vi "Results Status Update Process__core.vi"(8 "error in (no error)":errorcluster, 10 "TestRunner_UI_Refs":T2, 11 "TestStatusEvents":T1) -> (0 "error out":errorcluster)   [LabVIEW 2011, in "GraphicalTestRunner.lvlib"]
uses:
  GraphicalTestRunner.lvlib
  Classes/TestResult/resultStatus--enum.ctl
  Classes/TestSuite/suiteStatusChanged--Cluster.ctl
  Classes/TestSuite/suiteStatus--enum.ctl
  Classes/TestSuite/TestSuite.lvclass
  FailbarStatus--Enum.ctl
  Classes/TestResult/TestResult.lvclass
  <userlib>/_OpenG.lib/file/file.llb/Strip Path Extension - String__ogtk.vi
  Libraries/VITesterUtilities.lvlib
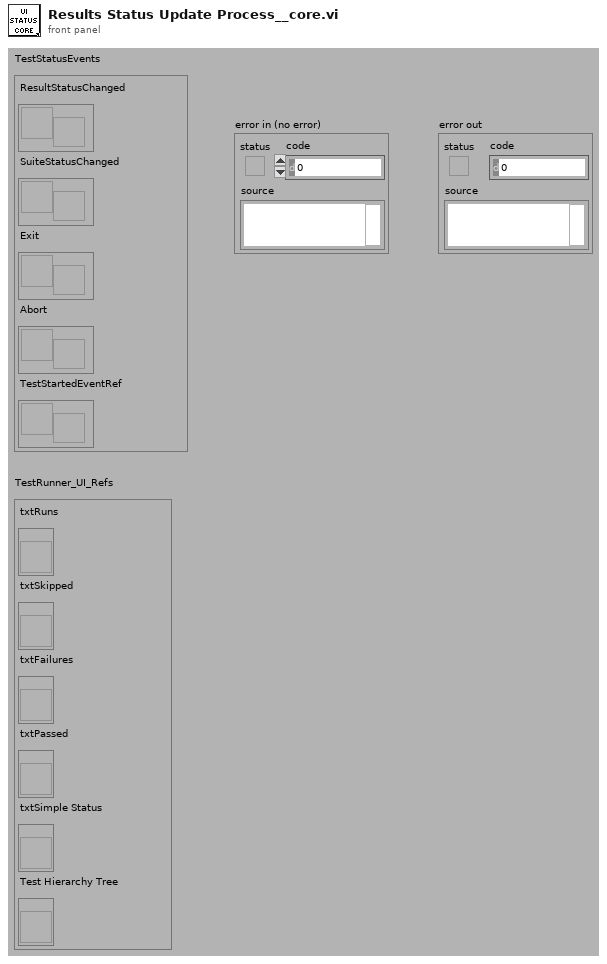
[diagram p1: front panel]
types:
  T1 = cluster{"ResultStatusChanged":refnum<user-event>, "SuiteStatusChanged":refnum<user-event>, "Exit":refnum<user-event>, "Abort":refnum<user-event>, "TestStartedEventRef":refnum<user-event>}
  T2 = cluster{"txtRuns":refnum<vi>, "txtSkipped":refnum<vi>, "txtFailures":refnum<vi>, "txtPassed":refnum<vi>, "txtSimple Status":refnum<vi>, "Test Hierarchy Tree":refnum<vi>}
  T3 = typedef "TestSuite.lvclass/suiteStatus--enum.ctl" = enum16{"suiteStart", "suiteStop", "suiteSkip"}
  T4 = typedef "GraphicalTestRunner.lvlib/FailbarStatus--Enum.ctl" = enum16{"Initialize", "Start", "Update Progress", "Fail", "Pass"}
  T5 = typedef "TestResult.lvclass/resultStatus--enum.ctl" = enum16{"testPass", "testFailure", "testError", "testSkipped"}
  T6 = typedef "TestResult.lvclass/failure.ctl" = cluster{"test":refnum<class>, "error":errorcluster}
  T7 = typedef "TestResult.lvclass/errors.ctl" = T8[]
  T8 = typedef "TestResult.lvclass/error.ctl" = cluster{"test":refnum<class>, "error":errorcluster}
  T9 = typedef "TestResult.lvclass/skipped.ctl" = T10[]
  T10 = typedef "TestResult.lvclass/skip.ctl" = cluster{"test":refnum<class>, "error":errorcluster}
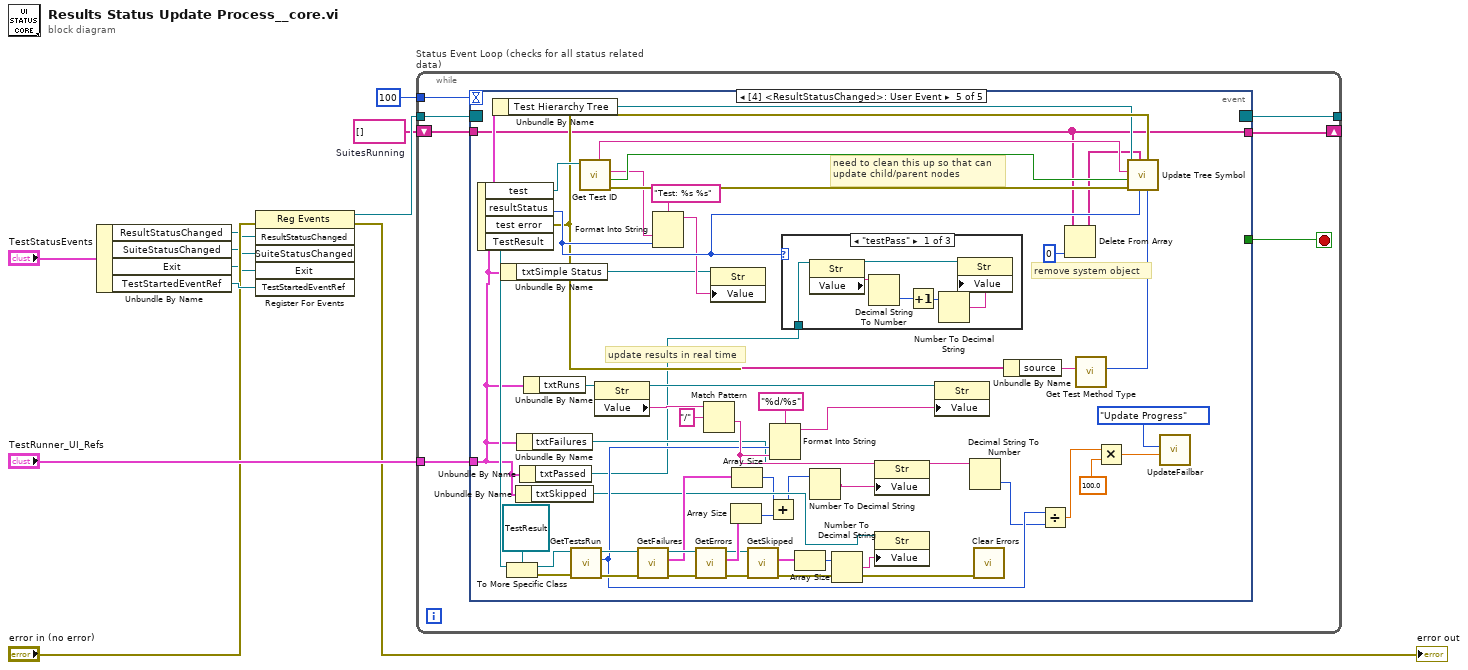
[diagram p0: block diagram]
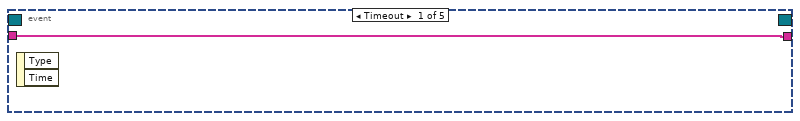
[diagram p2: hidden frame]
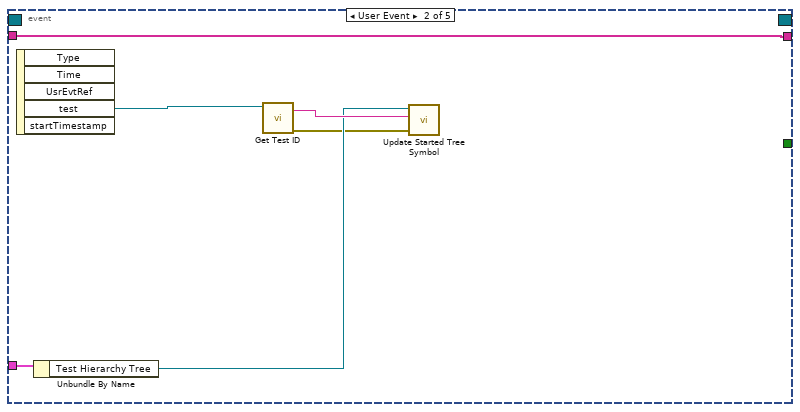
[diagram p3: hidden frame]
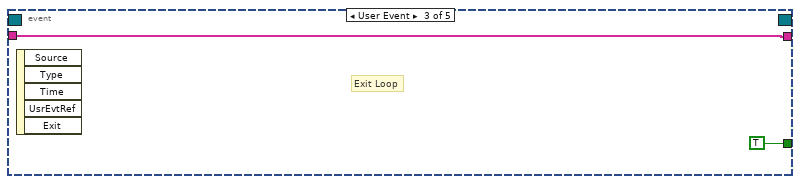
[diagram p4: hidden frame]
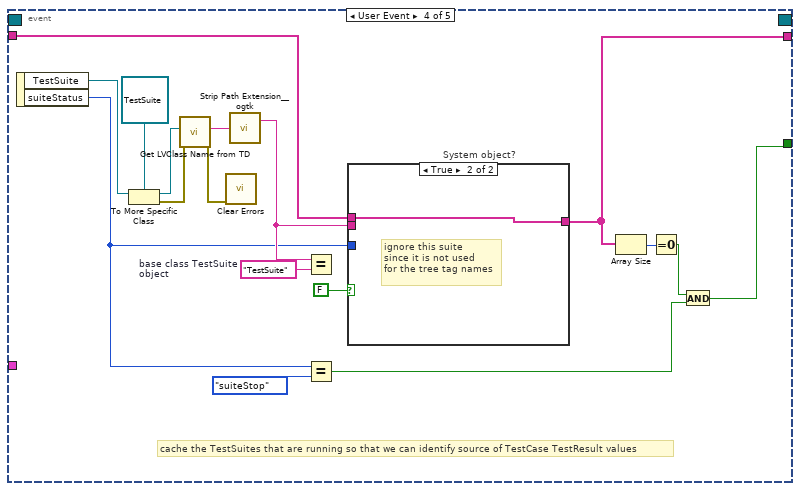
[diagram p5: hidden frame]
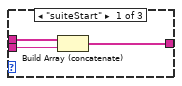
[diagram p7: hidden frame]
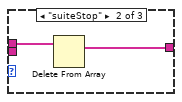
[diagram p8: hidden frame]
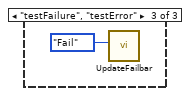
[diagram p10: hidden frame]
diagram:
  w1 = string[] []  # SuitesRunning
  n1 = Unbundle By Name("TestStatusEvents") -> ("ResultStatusChanged"=w5:refnum<user-event>, "SuiteStatusChanged"=w6:refnum<user-event>, "Exit"=w7:refnum<user-event>, "TestStartedEventRef"=w11:refnum<user-event>)
  n2 = register-events(error in="error in (no error)", w5, w6, w7, w11) -> (reference out=w3:refnum<event-registration>, error out=→"error out":errorcluster)  [unwired: 1 in]
  n3 = while "Status Event Loop (checks for all status related data)" {
    tunnel: w3 -> [w17]
    tunnel: [w16] -> _
    shift-right: [w14] -> _
    shift-left: w1 -> [w15]
    tunnel: 100 -> [w13]
    tunnel: "TestRunner_UI_Refs" -> [w12]
    stop <- w18 stop-if-true
    n4 = event shown="[4] <ResultStatusChanged>: User Event" {
      selector: w17 -> [_ _ _ _ _]
      dyn-events: [_ _ _ _ _] -> w16
      timeout: w13 -> [_ _ _ _ _]
      tunnel: [_ _ TRUE w29 _] -> w18
      tunnel: w15 -> [w19 w25 w27 w43 w60]
      tunnel: [w19 w25 w27 w35 w60] -> w14
      tunnel: w12 -> [_ w22 _ _ w65]
      event Timeout {
        n5 = event-data() -> ()  [unwired: 1 in, 2 out]
      }
      event User Event {
        n6 = event-data() -> ("test"=w24:refnum<class>)  [unwired: 1 in, 4 out]
        n7 = Unbundle By Name(w22) -> ("Test Hierarchy Tree"=w21:refnum<vi>)
        n8 = call "Get Test ID.vi"("Test In"=w24) -> ("error out"=w20:errorcluster, "GUID"=w23:string)  [unwired: 6 in, 3 out]
        n9 = call "Update Started Tree Symbol.vi"("error in"=w20, "test GUID"=w23, "Test Hierarchy Tree"=w21) -> ()  [unwired: 9 in]
      }
      event User Event {
        # "Exit Loop"
        n10 = event-data() -> ()  [unwired: 1 in, 5 out]
      }
      event User Event {
        w41 = "TestSuite"  # base class TestSuite object
        # "cache the TestSuites that are running so that we can identify source of TestCase TestResult values"
        n11 = event-data() -> ("TestSuite"=w39:refnum<class>, "suiteStatus"=w32:T3)  [unwired: 1 in]
        n12 = To More Specific Class(target class=refnum<class "TestSuite.lvclass"> refnum ("TestSuite.lvclass"), reference=w39) -> (specific class reference=w38:refnum<class "TestSuite.lvclass">, error out=w37:errorcluster)  [unwired: 1 in]
        n13 = call "Get LVClass Name from TD.vi"("error in"=w37, "Variant"=w38) -> ("error out"=w36:errorcluster, "LVClass Name"=w44:string)  [unwired: 8 in]
        n14 = call <vilib>:"Clear Errors.vi"("error in (no error)"=w36) -> ()  [unwired: 6 in, 1 out]
        n15 = call-poly <userlib>:"Strip Path Extension__ogtk.vi"("path"=w44) -> ("root"=w42:string)  [unwired: 1 out]
        n16 = Equal?(x=w42, y=w41) -> ()  [unwired: 1 out]
        n17 = Equal?(x=w32, y=suiteStatus--enum."suiteStop" ("suiteStatus")) -> (x = y?=w31:bool)
        n18 = case "System object?" shown="True" FALSE {
          tunnel: w32 -> [w48 _]
          tunnel: w43 -> [w47 w55]
          tunnel: w42 -> [w46 _]
          tunnel: [w45 w55] -> w35
          frame False {
            n19 = case shown="\"suiteSkip\"" w48 {
              tunnel: w47 -> [w51 w53 w54]
              tunnel: w46 -> [w50 _ _]
              tunnel: [w49 w52 w54] -> w45
              frame "suiteStart" {
                n20 = Build Array (concatenate)(w51, w50) -> (w49:string[])
              }
              frame "suiteStop" {
                n21 = Delete From Array(array=w53) -> (array with subset deleted=w52:string[])  [unwired: 2 in, 1 out]
              }
              frame "suiteSkip" {
                # "skip -don't update running\ntestSuites"
              }
            }
          }
          frame True {
            # "ignore this suite\nsince it is not used\nfor the tree tag names"
          }
        }
        n22 = Array Size(array=w35) -> (size(s)=w34:i32)
        n23 = Equal To 0?(x=w34) -> (x = 0?=w30:bool)
        n24 = And(x=w30, y=w31) -> (x .and. y?=w29:bool)
      }
      event User Event {
        # "remove system object"
        # "need to clean this up so that can\nupdate child/parent nodes"
        # "update results in real time"
        n25 = event-data() -> ("test"=w108:refnum<class>, "resultStatus"=w78:T5, "test error"=w77:errorcluster, "TestResult"=w99:refnum<class>)  [unwired: 1 in]
        n26 = Unbundle By Name(w65) -> ("Test Hierarchy Tree"=w66:refnum<vi>)
        n27 = Unbundle By Name(w65) -> ("txtSimple Status"=w63:refnum<vi>)
        n28 = To More Specific Class(target class=refnum<class "TestResult.lvclass"> refnum ("reference in"), reference=w99) -> (specific class reference=w98:refnum<class "TestResult.lvclass">, error out=w94:errorcluster)  [unwired: 1 in]
        n29 = Unbundle By Name(w65) -> ("txtSkipped"=w67:refnum<vi>)
        n30 = Unbundle By Name(w65) -> ("txtFailures"=w70:refnum<vi>)
        n31 = Unbundle By Name(w65) -> ("txtPassed"=w59:refnum<vi>)
        n32 = Unbundle By Name(w65) -> ("txtRuns"=w74:refnum<vi>)
        n33 = call-dynamic "GetTestsRun.vi"("error in (no error)"=w94, "TestResult in"=w98) -> ("error out"=w104:errorcluster, "testsRun"=w91:u32, "TestResult out"=w106:refnum<class "TestResult.lvclass">)  [unwired: 7 in]
        n34 = call "Get Test ID.vi"("Test In"=w108) -> ("error out"=w95:errorcluster, "IsTestCase"=w81:bool, "id"=w76:string, "GUID"=w75:string)  [unwired: 6 in, 1 out]
        n35 = property class="Str"(reference=w74) -> (reference out=w71:refnum<vi>, "Value"=w73:string)  [unwired: 1 in, 1 out]
        n36 = call-dynamic "GetFailures.vi"("error in (no error)"=w104, "TestResult in"=w106) -> ("error out"=w103:errorcluster, "failures"=w101:T6[], "TestResult out"=w105:refnum<class "TestResult.lvclass">)  [unwired: 7 in]
        n37 = Format Into String(format string="Test: %s %s", w76, w78) -> (resulting string=w64:string)  [unwired: 2 in, 1 out]
        n38 = call-dynamic "GetErrors.vi"("error in (no error)"=w103, "TestResult in"=w105) -> ("error out"=w86:errorcluster, "Errors"=w102:T7, "TestResult out"=w85:refnum<class "TestResult.lvclass">)  [unwired: 7 in]
        n39 = Match Pattern(string=w73, regular expression="/") -> (after substring=w92:string)  [unwired: 1 in, 3 out]
        n40 = property class="Str"(reference=w63, "Value"=w64) -> ()  [unwired: 1 in, 2 out]
        n41 = Array Size(array=w102) -> (size(s)=w58:i32)
        n42 = Array Size(array=w101) -> (size(s)=w57:i32)
        n43 = call-dynamic "GetSkipped.vi"("error in (no error)"=w86, "TestResult in"=w85) -> ("error out"=w82:errorcluster, "Skipped"=w83:T9)  [unwired: 7 in, 1 out]
        n44 = Add(x=w57, y=w58) -> (x+y=w56:i32)
        n45 = Format Into String(format string="%d/%s", w91, w92) -> (resulting string=w72:string)  [unwired: 2 in, 1 out]
        n46 = case shown="\"testPass\"" w78 {
          tunnel: w59 -> [w114 _ _]
          frame "testPass" {
            n47 = property class="Str"(reference=w114) -> (reference out=w111:refnum<vi>, "Value"=w113:string)  [unwired: 1 in, 1 out]
            n48 = Decimal String To Number(string=w113) -> (number=w112:i32)  [unwired: 2 in, 1 out]
            n49 = Increment(x=w112) -> (x+1=w110:i32)
            n50 = Number To Decimal String(number=w110) -> (decimal integer string=w109:string)  [unwired: 1 in]
            n51 = property class="Str"(reference=w111, "Value"=w109) -> ()  [unwired: 1 in, 2 out]
          }
          frame "testSkipped" {
          }
          frame "testFailure", "testError" {
            n52 = call "UpdateFailbar.vi"("Function"=FailbarStatus--Enum."Fail") -> ()  [unwired: 11 in]
          }
        }
        n53 = Array Size(array=w83) -> (size(s)=w84:i32)
        n54 = Number To Decimal String(number=w56) -> (decimal integer string=w69:string)  [unwired: 1 in]
        n55 = Number To Decimal String(number=w84) -> (decimal integer string=w68:string)  [unwired: 1 in]
        n56 = property class="Str"(reference=w70, "Value"=w69) -> ()  [unwired: 1 in, 2 out]
        n57 = property class="Str"(reference=w67, "Value"=w68) -> ()  [unwired: 1 in, 2 out]
        n58 = property class="Str"(reference=w71, "Value"=w72) -> ()  [unwired: 1 in, 2 out]
        n59 = Decimal String To Number(string=w92) -> (number=w90:i32)  [unwired: 2 in, 1 out]
        n60 = call <vilib>:"Clear Errors.vi"("error in (no error)"=w82) -> ()  [unwired: 6 in, 1 out]
        n61 = Unbundle By Name(w77) -> ("source"=w80:string)
        n62 = Divide(x=w91, y=w90) -> (x/y=w89:dbl)
        n63 = Delete From Array(array=w60, index=0) -> (array with subset deleted=w61:string[])  [unwired: 1 in, 1 out]
        n64 = call "Get Test Method Type.vi"("Failure String"=w80) -> ("method type"=w79:enum16{"setUp", "testMethod", "tearDown"})  [unwired: 10 in]
        n65 = Multiply(x=w89, y=100.0) -> (x*y=w88:dbl)
        n66 = call "Update Tree Symbol.vi"("method type"=w79, "test error"=w77, "resultStatus"=w78, "SuitesRunning"=w61, "error in"=w95, "IsTestCase"=w81, "test GUID"=w75, "Test Hierarchy Tree"=w66) -> ()  [unwired: 4 in]
        n67 = call "UpdateFailbar.vi"("Progress"=w88, "Function"=FailbarStatus--Enum."Update Progress") -> ()  [unwired: 10 in]
      }
    }
  }
